vi "Write jav rad.vi"(8 "error in (no error)":errorcluster, 10 "jav rad":dbl[](array[numeric])=[0.15, 0.15, 0.25], 11 "Constant Jerk Guidance in":refnum<class "Constant Jerk Guidance.lvclass">) -> (0 "error out":errorcluster, 3 "Constant Jerk Guidance out":refnum<class "Constant Jerk Guidance.lvclass">)   [LabVIEW 2014, in "Guidance Library.lvlib" / "Constant Jerk Guidance.lvclass"]
uses:
  Constant Jerk Guidance.lvclass
  Constant Jerk Guidance.lvclass/Constant Jerk Guidance.ctl
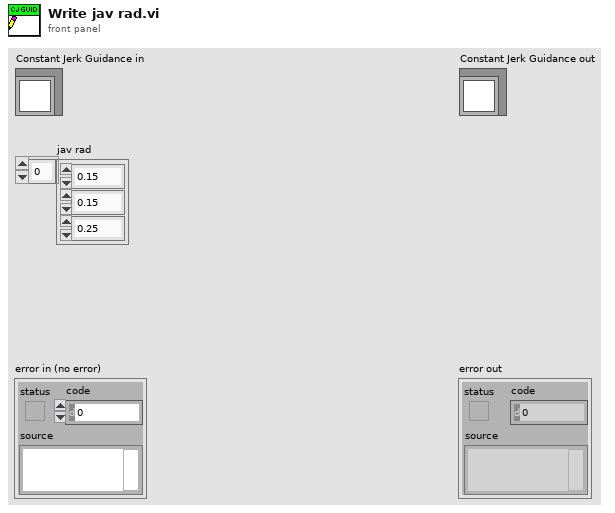
[diagram p1: front panel]
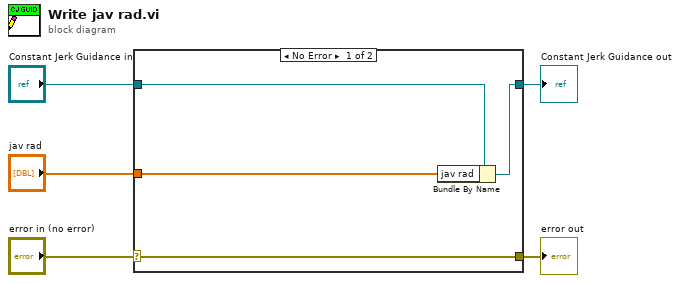
[diagram p0: block diagram]
diagram:
  n1 = case shown="No Error" "error in (no error)" {
    selector: "error in (no error)" -> [w9 w10]
    tunnel: [w9 w10] -> w4
    tunnel: [w7 w11] -> w2
    tunnel: "Constant Jerk Guidance in" -> [w8 w11]
    tunnel: "jav rad" -> [w6 _]
    frame No Error {
      n2 = Bundle By Name(cluster=w8, "jav rad"=w6) -> (w7:refnum<class "Constant Jerk Guidance.lvclass">)
    }
    frame Error {
    }
  }
  "error out" <- w4
  "Constant Jerk Guidance out" <- w2
